vi "invert.vi"() -> ()   [LabVIEW 2017]
uses:
  <vilib>/Analysis/NI_AALBase.lvlib
panel:
  out "Waveform Graph":waveform(dbl)(graph)
  in  "invert":bool
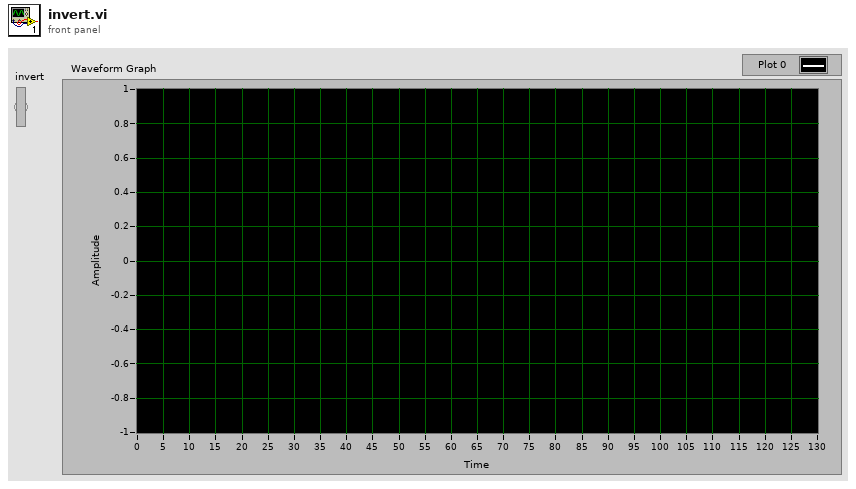
[diagram p1: front panel]
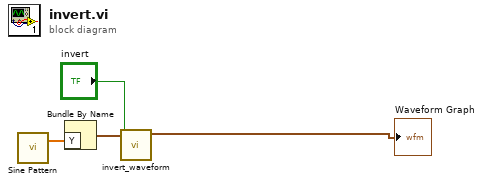
[diagram p0: block diagram]
diagram:
  n1 = call <vilib>:"Sine Pattern.vi"() -> ("Sinusoidal Pattern"=w4:dbl[])  [unwired: 4 in, 1 out]
  n2 = Bundle By Name("Y"=w4) -> (w3:waveform(dbl))  [unwired: 1 in]
  n3 = call "invert_waveform.vi"("invert"="invert", "waveform"=w3) -> ("output waveform"=→"Waveform Graph":waveform(dbl))  [unwired: 9 in]
